vi "Create Queues.vi"(8 "error in (no error)":errorcluster, 11 "GenBus_Load_Calculator in":refnum<class "CANBus_Load_Calculator.lvclass">) -> (0 "error out":errorcluster, 3 "GenBus_Load_Calculator out":refnum<class "CANBus_Load_Calculator.lvclass">)   [LabVIEW 2018, in "NI-XNET Monitor Engine.lvlib" / "XNET-Bus-Load-Calculator.lvlib" / "CANBus_Load_Calculator.lvclass"]
uses:
  CANBus_Load_Calculator.lvclass
  typedefs/ToCalculator_Data.ctl
  typedefs/FromCalculator_Data.ctl
  CANBus_Load_Calculator.lvclass/CANBus_Load_Calculator.ctl
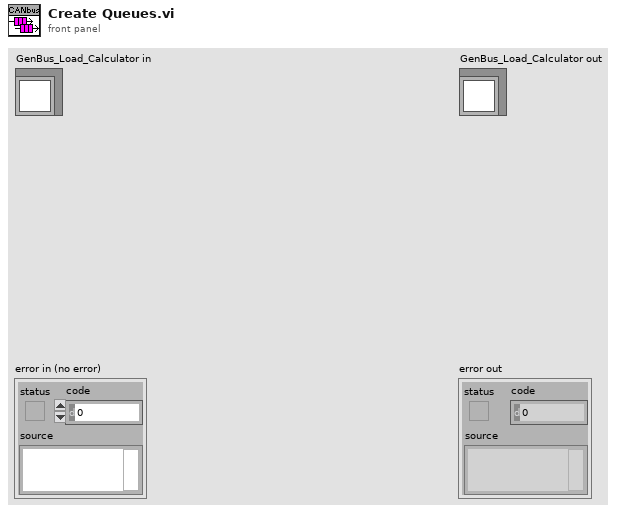
[diagram p1: front panel]
types:
  T1 = typedef "NI-XNET Monitor Engine.lvlib/XNET-Bus-Load-Calculator.lvlib/CANBus_Load_Calculator.lvclass/FromCalculator_Data.ctl" = cluster{"Bus Load (%)":dbl}
  T2 = typedef "NI-XNET Monitor Engine.lvlib/XNET-Bus-Load-Calculator.lvlib/CANBus_Load_Calculator.lvclass/ToCalculator_Data.ctl" = cluster{"Stop":bool, "Bus Busy Time (us)":u64}
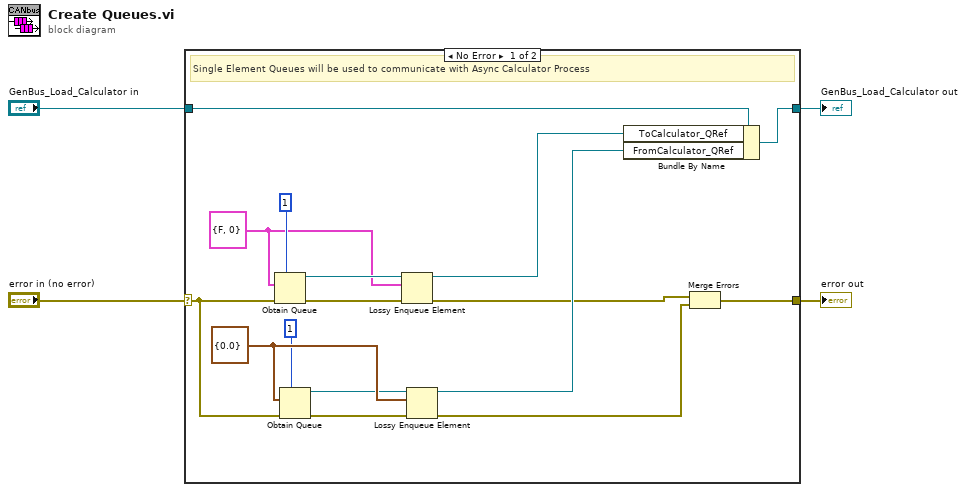
[diagram p0: block diagram]
diagram:
  n1 = case shown="No Error" "error in (no error)" {
    selector: "error in (no error)" -> [w9 w22]
    tunnel: [w5 w22] -> w3
    tunnel: [w19 w21] -> w1
    tunnel: "GenBus_Load_Calculator in" -> [w20 w21]
    frame No Error {
      w13 = T1 {"Bus Load (%)"=0.0} ("FromCalculator_Data")
      w15 = T2 {"Stop"=FALSE, "Bus Busy Time (us)"=0} ("ToCalculator_Data")
      # "Single Element Queues will be used to communicate with Async Calculator Process"
      n2 = Obtain Queue(max queue size (-1, unlimited)=1, element data type=w15, error in (no error)=w9) -> (queue out=w16:refnum<queue>, error out=w17:errorcluster)  [unwired: 2 in, 1 out]
      n3 = Obtain Queue(max queue size (-1, unlimited)=1, element data type=w13, error in (no error)=w9) -> (queue out=w12:refnum<queue>, error out=w11:errorcluster)  [unwired: 2 in, 1 out]
      n4 = Lossy Enqueue Element(queue=w16, element=w15, error in (no error)=w17) -> (queue out=w14:refnum<queue>, error out=w7:errorcluster)  [unwired: 2 out]
      n5 = Lossy Enqueue Element(queue=w12, element=w13, error in (no error)=w11) -> (queue out=w8:refnum<queue>, error out=w6:errorcluster)  [unwired: 2 out]
      n6 = Bundle By Name(cluster=w20, "ToCalculator_QRef"=w14, "FromCalculator_QRef"=w8) -> (w19:refnum<class "CANBus_Load_Calculator.lvclass">)
      n7 = Merge Errors(w7, w6) -> (w5:errorcluster)
    }
    frame Error {
    }
  }
  "error out" <- w3
  "GenBus_Load_Calculator out" <- w1
